vi "deinitialize.vi"(0 "NInstrSim":refnum<class "NInstrSim.lvclass">, 5 "error in (no error)":errorcluster) -> (19 "error out":errorcluster)   [LabVIEW 2009, in "HB_Device_Examples.lvlib" / "NInstrSim.lvclass"]
doc: "This is a dynamic dispatch VI. It can be overwritten by childclasses to release allocated recources."
uses:
  NInstrSim.lvclass
  lib.lib/HGF_LVC/HGF_DeviceBaseClasses/HGF_VISADevice/HGF_VISADevice.lvclass
  non_GPL/instr.lib/NI Instrument Simulator/NI Instrument Simulator.lvlib
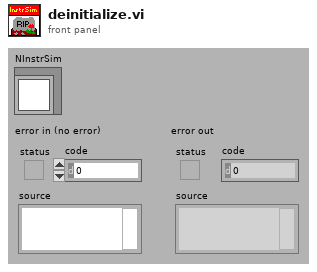
[diagram p1: front panel]
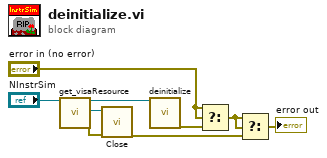
[diagram p0: block diagram]
diagram:
  n1 = call "get_visaResource.vi"("HGF_VISADevice"="NInstrSim") -> ("dup HGF_VISADevice"=w8:refnum<class "NInstrSim.lvclass">, "VISA Resource Name"=w7:refnum<visa-resource-name>, "error out"=w6:errorcluster)  [unwired: 1 in, 15 out]
  n2 = call "Close.vi"("error in (no error)"=w6, "VISA resource name"=w7) -> ("error out"=w2:errorcluster)  [unwired: 9 out]
  n3 = call-parent "deinitialize.vi"("HGF_DeviceBase"=w8) -> ("error out"=w4:errorcluster)  [unwired: 1 in, 17 out]
  n4 = Select(t="error in (no error)", s="error in (no error)", f=w4) -> (s? t:f=w3:errorcluster)
  n5 = Select(t=w3, s=w3, f=w2) -> (s? t:f=→"error out":errorcluster)
